vi "Parse State Queue_csmlite.vi"(0 "State Queue":string, 1 "Current Module(\"\" to generate an ID)":string="Debug-LogViewer", 7 "Error In (no error)":errorcluster) -> (3 "Event Registration Refnum":refnum<event-registration>, 4 "Remaining States":string, 6 "Current State":string, 8 "Arguments":string)   [LabVIEW 2017, in "_csmlite.lvlib"]
doc: "Parses the JKI State Machine state queue and returns the current state that will execute next with the associated arguments.\n\nFor instructions on how to use the JKI State Machine, examples and video tutorials, visit:\nhttp://jkisoft.com/state-machine/\n\n<B>Inputs:</B>\n <B>State Queue:</B> The entire state queue is wired to this input. This should come from the main JKI State Machine shift register.\n <B>Error In</B> The error cluster from the JKI State Machine is wired to this input. If an error occures and appears on this input, the current state output returns the \"Error Handler\" state.\n\n<B>Outputs:</B>\n <B>Remaining States:</B> Returns all the next states that should execute after the current state completes. These should be passed through the current state in the state machine. These can also be modified or augmented within the current state if necessary.\n <B>Current State:</B> Returns the current state that should execute next in the state machine. If an error is wired to the Error input then the current state output becomes \"Error Handler\".\n <B>Arguments:</B> Returns any argument(s) that may be used in the current state string. These arguments come after the \">>\" characters. <B>Note:</B> The arguments variable must not contain any unprintable characters like linefeed or carriage return.\n\n<B>State Syntax:</B>\nStateCategory: State >> Argument\nLine Terminator: Line feed\n <B>Example:</B>\nUI: Help >> About\n\nWhere \"UI\" is the state category\nWhere \"Help\" is the state\nWhere \"About\" is the argument\n <B>Other Examples:</B>\nApp Data: Initialize\nUI: Initialize\nHelp >> About\n\n<B>Commenting:</B>\nTo add a comment use \"//\" or \"#\" and all text to the right will be ignored\n <B>Commenting Example:</B>\nUI: Initialize // This initializes the UI\n# This whole line is a comment\n// Another comment line\n\nJKI State Machine™ 2018.0.7.45\nhttp://jki.net/state-machine/\nCopyright (C) 2005-2018, JKI <info@jki.net>\nALL RIGHTS RESERVED"
uses:
  _csmlite.lvlib
  _action.ctl
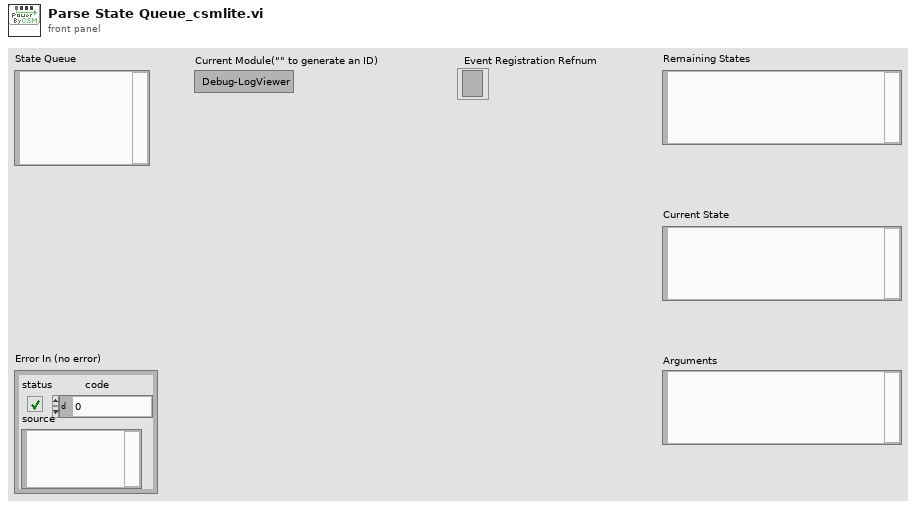
[diagram p1: front panel]
types:
  T1 = typedef "_csmlite.lvlib/_action.ctl" = enum16{"Obtain", "Destroy", "Broadcast", "Post"}
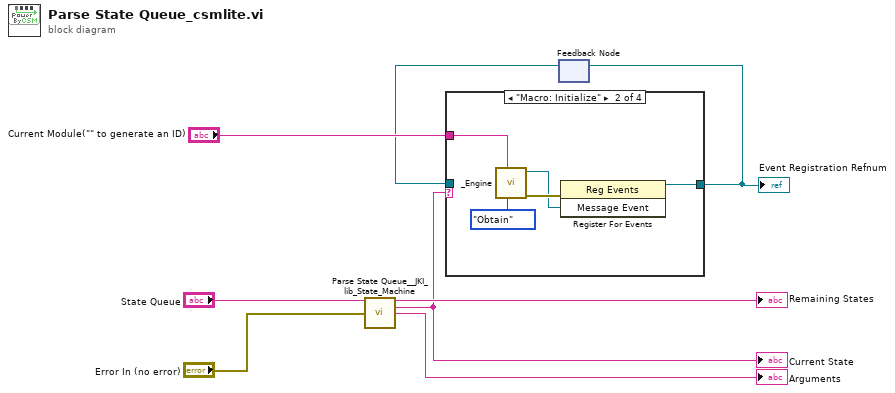
[diagram p0: block diagram]
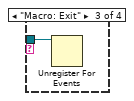
[diagram p3: hidden frame]
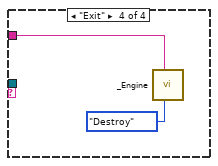
[diagram p4: hidden frame]
diagram:
  n1 = call <vilib>:"Parse State Queue__JKI_lib_State_Machine.vi"("State Queue"="State Queue", "Error In (no error)"="Error In (no error)") -> ("Remaining States"=→"Remaining States":string, "Current State"=w3:string, "Arguments"=→"Arguments":string)  [unwired: 11 in]
  "Current State" <- w3
  n2 = feedback #1() -> (w2:refnum<event-registration>)  [unwired: 1 in]
  n3 = case shown="\"Macro: Initialize\"" w3 {
    tunnel: "Current Module(\"\" to generate an ID)" -> [_ w12 _ w16]
    tunnel: [w9 w11 _ _] -> w1
    tunnel: w2 -> [w9 _ w15 _]
    frame "False", Default {
    }
    frame "Macro: Initialize" {
      n4 = call "_Engine.vi"("Enum"=_action."Obtain", "Module Name"=w12) -> ("Error out"=w14:errorcluster, "Message Event"=w10:refnum<user-event>)  [unwired: 8 in]
      n5 = register-events(error in=w14, w10) -> (reference out=w11:refnum<event-registration>)  [unwired: 1 in, 1 out]
    }
    frame "Macro: Exit" {
      n6 = Unregister For Events(event registration refnum=w15) -> ()  [unwired: 1 in, 1 out]
    }
    frame "Exit" {
      n7 = call "_Engine.vi"("Enum"=_action."Destroy", "Module Name"=w16) -> ()  [unwired: 8 in, 2 out]
    }
  }
  "Event Registration Refnum" <- w1
  n8 = feedback-in #1(w1) -> ()
